vi "Sensor_Impluse.vi"() -> ()   [LabVIEW 2018]
panel:
  out "Impulse(J)":dbl[](array[numeric])
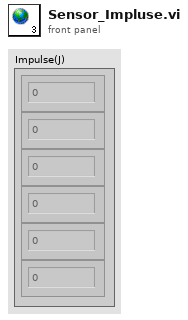
[diagram p1: front panel]
diagram:
